vi "Go to LeafNode.vi"(8 "error in":errorcluster caption="错误输入（无错误）", 10 "LeafNumber":string, 11 "PanelRootNode 输入":refnum<class "PanelRootNode.lvclass"> caption="DNL_LabVIEW Object in") -> (0 "error out":errorcluster caption="错误输出", 1 "is rootnode?":bool, 2 "Node*":refnum<data-value>, 3 "PanelRootNode 输出":refnum<class "PanelRootNode.lvclass"> caption="DNL_LabVIEW Object out")   [LabVIEW 2016, in "PanelRootNode.lvclass"]
uses:
  PanelRootNode.lvclass
  PanelObject/PanelObject.lvclass
  PanelRootNode.lvclass/PanelRootNode.ctl
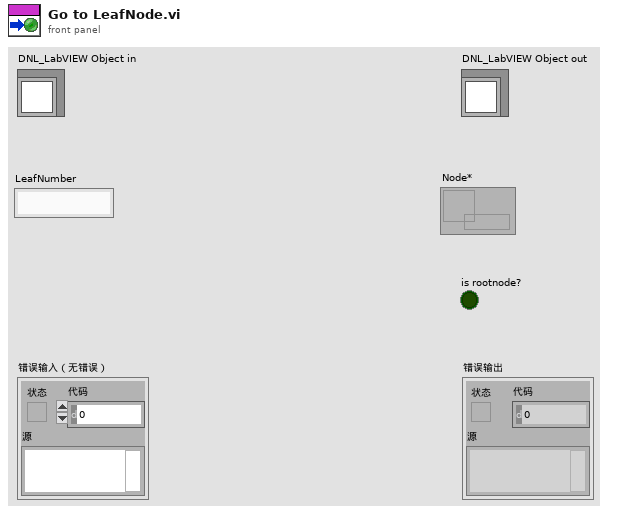
[diagram p1: front panel]
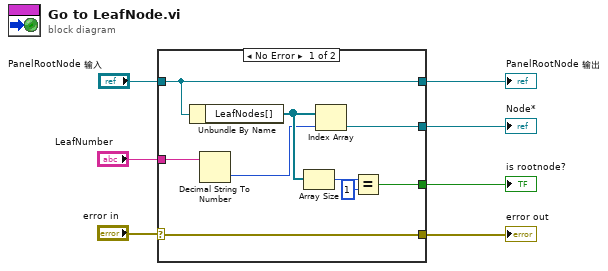
[diagram p0: block diagram]
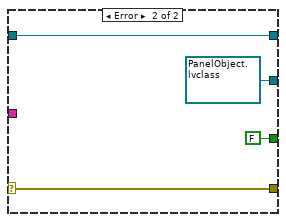
[diagram p2: hidden frame]
diagram:
  n1 = case shown="No Error" "error in" {
    selector: "error in" -> [w9 w17]
    tunnel: "PanelRootNode 输入" -> [w16 w20]
    tunnel: "LeafNumber" -> [w15 _]
    tunnel: [w16 w20] -> w4
    tunnel: [w14 refnum<data-value> refnum ("Node*")] -> w3
    tunnel: [w10 FALSE] -> w2
    tunnel: [w9 w17] -> w1
    frame No Error {
      n2 = Unbundle By Name(w16) -> ("LeafNodes[]"=w13:refnum<data-value>[])
      n3 = Decimal String To Number(string=w15) -> (number=w8:i32)  [unwired: 2 in, 1 out]
      n4 = Array Size(array=w13) -> (size(s)=w12:i32)
      n5 = Index Array(array=w13, index=w8) -> (element=w14:refnum<data-value>)
      n6 = Equal?(x=w12, y=1) -> (x = y?=w10:bool)
    }
    frame Error {
    }
  }
  "error out" <- w1
  "PanelRootNode 输出" <- w4
  "is rootnode?" <- w2
  "Node*" <- w3
